vi "Benchmark SV Receive LV2012 - NI Verified - 100 Byte.vi"() -> ()   [LabVIEW 2015]
panel:
  out "appended array":i32[][](array[numeric])
  in  "100 byte 2":i32[][](array[numeric])=[[0, 0, 0, 0, 0, 0, 0, 0, 0, 0], [0, 0, 0, 0, 0, 0, 0, 0, 0, 0], [0, 0, 0, 0, 0, 0, 0, 0, 0, 0], [0, 0, 0, 0, 0, 0, 0, 0, 0, 0], [0, 0, 0, 0, 0, 0, 0, 0, 0, 0], [0, 0, 0, 0, 0, 0, 0, 0, 0, 0], [0, 0, 0, 0, 0, 0, 0, 0, 0, 0], [0, 0, 0, 0, 0, 0, 0, 0, 0, 0], [0, 0, 0, 0, 0, 0, 0, 0, 0, 0], [0, 0, 0, 0, 0, 0, 0, 0, 0, 0]]
  out "100 byte":i32[][](array[numeric])
  in  "stop":bool
  # "Overview:  Coding that exemplifies how to benchmark the communication of Shared Variables.\nRequirements: LabVIEW 2012 or compatible\nInstructions:\n1. Run this VI\n2. Watch the amount of time it takes to communicate on the \"Benchmark SV Send  LV2012 - NI Verified.vi\" \n3. Stop both VIs"
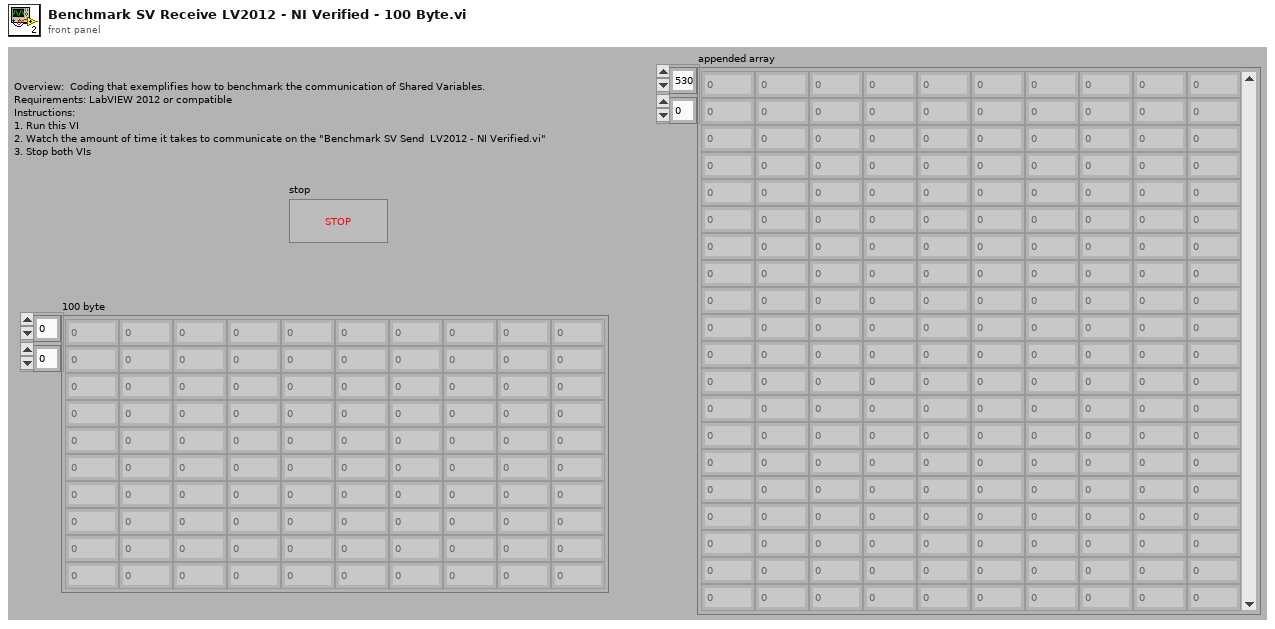
[diagram p1: front panel]
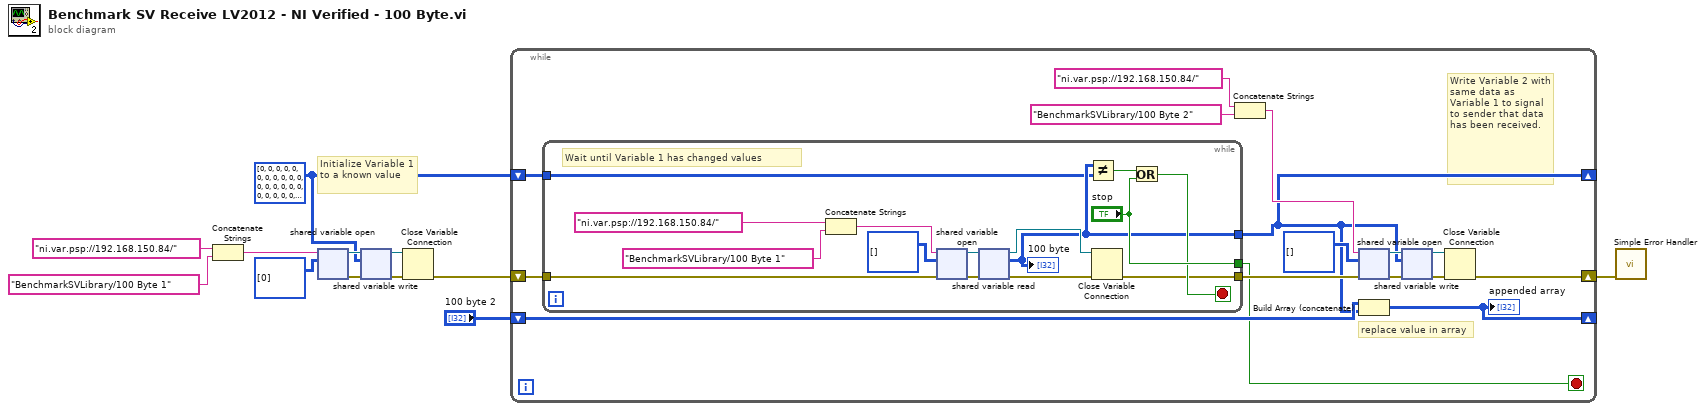
[diagram p0: block diagram]
diagram:
  w1 = i32[][] [[0, 0, 0, 0, 0, 0, 0, 0, 0, 0], [0, 0, 0, 0, 0, 0, 0, 0, 0, 0], [0, 0, 0, 0, 0, 0, 0, 0, 0, 0], [0, 0, 0, 0, 0, 0, 0, 0, 0, 0], [0, 0, 0, 0, 0, 0, 0, 0, 0, 0], [0, 0, 0, 0, 0, 0, 0, 0, 0, 0], [0, 0, 0, 0, 0, 0, 0, 0, 0, 0], [0, 0, 0, 0, 0, 0, 0, 0, 0, 0], [0, 0, 0, 0, 0, 0, 0, 0, 0, 0], [0, 0, 0, 0, 0, 0, 0, 0, 0, 0]] ("appended array")
  # "Initialize Variable 1 to a known value"
  n1 = Concatenate Strings("ni.var.psp://192.168.150.84/" ("string"), "BenchmarkSVLibrary/100 Byte 1") -> (w11:string)
  n2 = shared-variable-open(w11, i32[][] [[0]] ("appended array")) -> (w9:refnum<k21>, w7:errorcluster)  [unwired: 2 in]
  n3 = shared-variable-write(w9, w7, w1) -> (w8:refnum<k21>, w6:errorcluster)
  n4 = Close Variable Connection(8:w6, 11:w8) -> (0:w5:errorcluster)
  n5 = while {
    shift-right: [w18] -> w12
    shift-left: w5 -> [w28]
    shift-right: [w17] -> _
    shift-left: "100 byte 2" -> [w15]
    shift-right: [w14] -> _
    shift-left: w1 -> [w16]
    stop <- w13 stop-if-true
    # "replace value in array"
    # "Write Variable 2 with same data as Variable 1 to signal to sender that data has been received."
    n6 = while {
      tunnel: [w30] -> w14
      tunnel: ["stop"] -> w13
      tunnel: [w35] -> w19
      tunnel: w28 -> [w34]
      tunnel: w16 -> [w29]
      stop <- w41 stop-if-true
      # "Wait until Variable 1 has changed values"
      n7 = Concatenate Strings("ni.var.psp://192.168.150.84/" ("string"), "BenchmarkSVLibrary/100 Byte 1") -> (w31:string)
      n8 = shared-variable-open(w31, w34, i32[][] [] ("appended array")) -> (w39:refnum<k21>, w38:errorcluster)  [unwired: 1 in]
      n9 = shared-variable-read(w39, w38) -> (w37:refnum<k21>, w36:errorcluster, w30:i32[][])  [unwired: 1 out]
      "100 byte" <- w30
      n10 = Not Equal?(x=w30, y=w29) -> (x != y?=w43:bool)
      n11 = Close Variable Connection(8:w36, 11:w37) -> (0:w35:errorcluster)
      n12 = Or(x=w43, y="stop") -> (x .or. y?=w41:bool)
    }
    n13 = Concatenate Strings("ni.var.psp://192.168.150.84/" ("string"), "BenchmarkSVLibrary/100 Byte 2") -> (w26:string)
    n14 = shared-variable-open(w26, w19, i32[][] [] ("appended array")) -> (w25:refnum<k21>, w24:errorcluster)  [unwired: 1 in]
    n15 = Build Array (concatenate)(w15, w14) -> (w17:i32[][])
    "appended array" <- w17
    n16 = shared-variable-write(w25, w24, w14) -> (w23:refnum<k21>, w22:errorcluster)
    n17 = Close Variable Connection(8:w22, 11:w23) -> (0:w18:errorcluster)
  }
  n18 = call <vilib>:"Simple Error Handler.vi"("error in (no error)"=w12) -> ()  [unwired: 4 in, 5 out]
